vi "Write SCPI Command.vi"(8 "error in (no error)":errorcluster, 10 "SCPI Command":string, 11 "36234A in":refnum<class "36234A.lvclass">) -> (0 "error out":errorcluster, 3 "36234A out":refnum<class "36234A.lvclass">)   [LabVIEW 2019, in "36234A.lvlib" / "36234A.lvclass"]
uses:
  Library/36234A.lvclass
  Library/36234A.lvclass/36234A.ctl
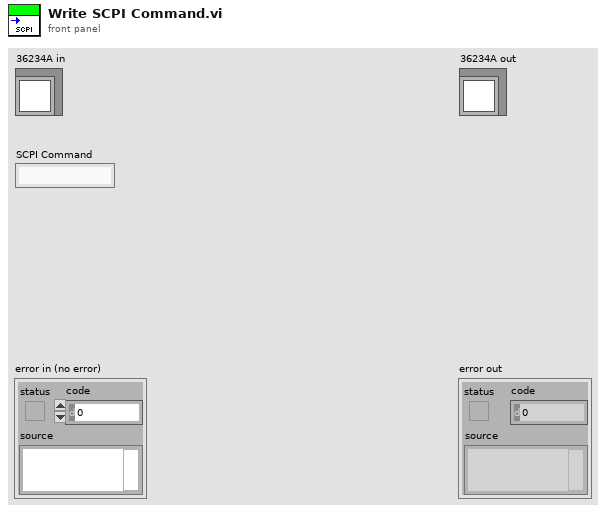
[diagram p1: front panel]
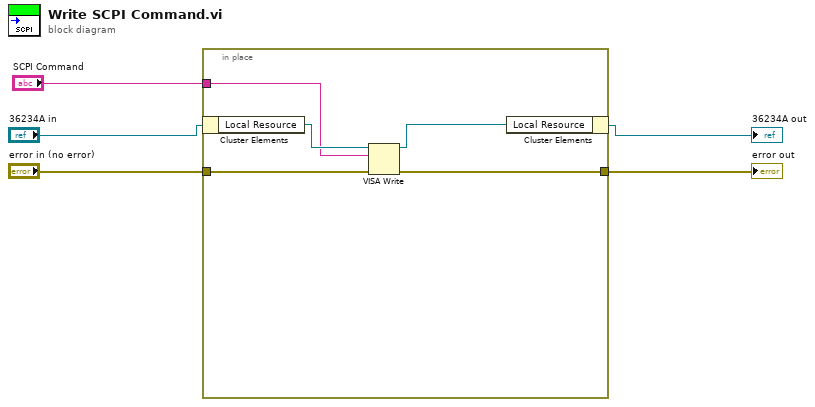
[diagram p0: block diagram]
diagram:
  n1 = in-place {
    in-place-border: [w8] -> w3
    in-place-border: "error in (no error)" -> [w7]
    in-place-border: "SCPI Command" -> [w6]
    n2 = in-place-cluster #1("36234A in") -> ("Local Resource"=w10:refnum<visa-resource-name>)
    n3 = VISA Write(VISA resource name=w10, write buffer=w6, error in (no error)=w7) -> (VISA resource name out=w9:refnum<visa-resource-name>, error out=w8:errorcluster)  [unwired: 1 out]
    n4 = in-place-cluster #1("Local Resource"=w9) -> (→"36234A out":refnum<class "36234A.lvclass">)
  }
  "error out" <- w3
